vi "Write_ERD_Data_to_File.vi"(0 "refnum in":refnum<file>, 1 "ERD_Always Show":T6, 5 "Redundant Micro":T4, 7 "Version":T5, 9 "ERD Graph  Ind 2":T3, 11 "Error In":errorcluster, 12 "ATC Data":T2, 13 "Algorithm Data":T1) -> (4 "refnum out":refnum<file>, 15 "Error Out":errorcluster)   [LabVIEW 2014]
uses:
  type defs/ERD_Always_Show.ctl
  type defs/Version.ctl
  type defs/Redundant.ctl
  type defs/ATC_Data.ctl
  type defs/Algorithms.ctl
panel:
  # "Wet Load Size"
  # "Dry Load Size"
  # "OOB"
  # "Software Version"
  # "Critical Version"
  # "Non-Critical"
  # "XML Crit Ver"
  # "XML Non-Crit"
  # "Daily Build"
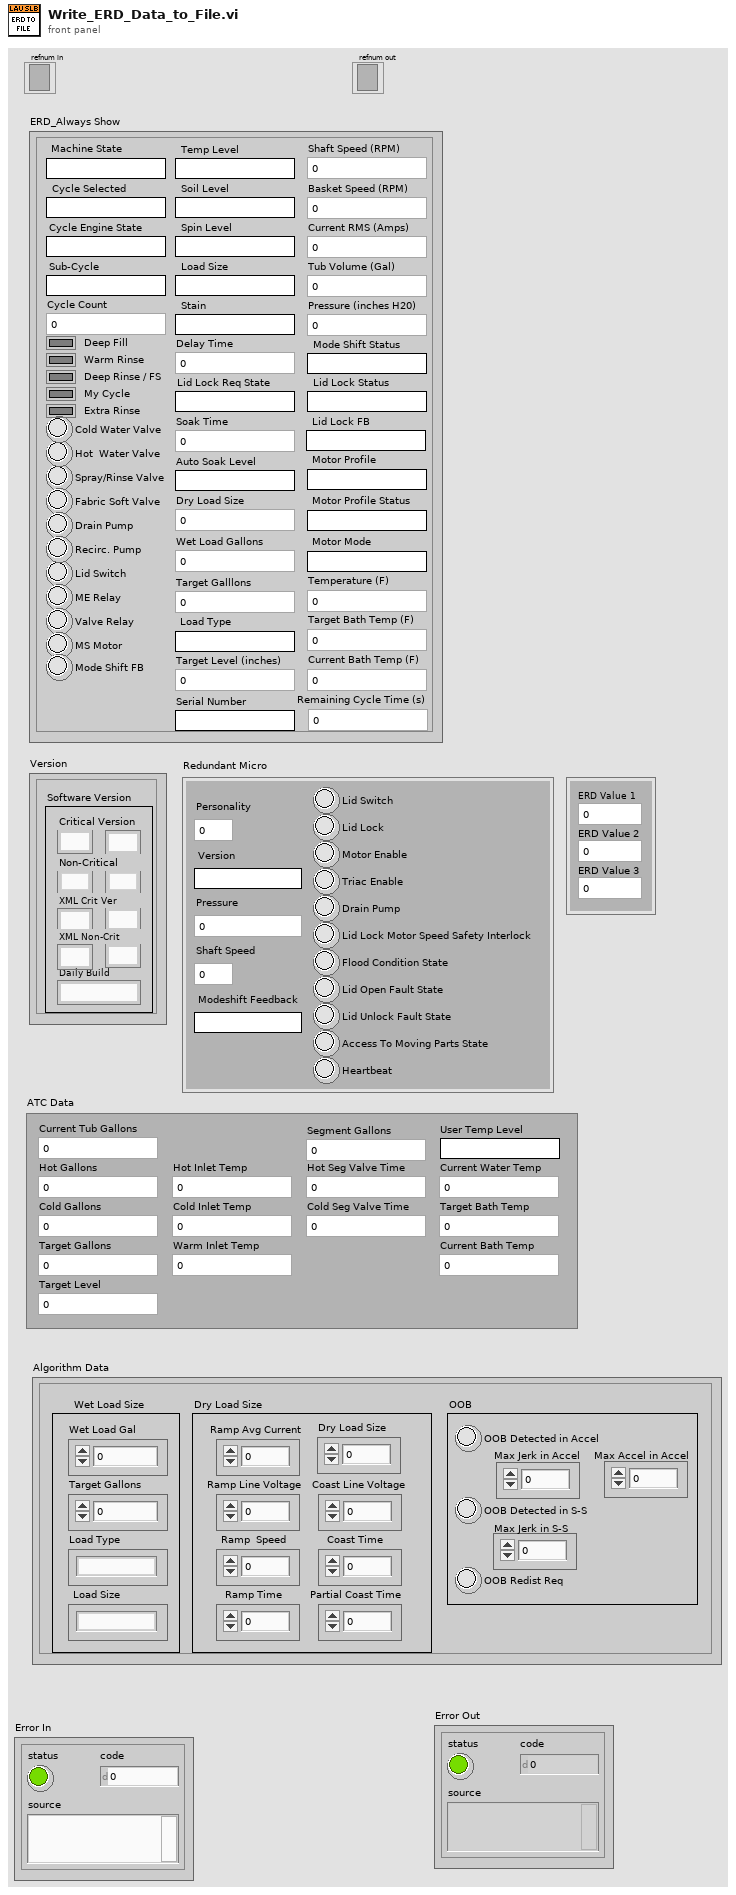
[diagram p1: front panel]
types:
  T1 = typedef "Algorithms.ctl" = cluster{"Wet Load Gal":dbl, "Target Gallons":dbl, "Load Type":string, "Load Size":string, "Coast Time":u16, "Ramp Time":u16, "Ramp  Speed":u16, "Ramp Avg Current":dbl, "OOB Redist Req":bool, "OOB Detected in S-S":bool, "Max Accel in Accel":i32, "Max Jerk in Accel":i32, "Max Jerk in S-S":i32, "OOB Detected in Accel":bool, "Partial Coast Time":u16, "Dry Load Size":dbl, "Ramp Line Voltage ":dbl, "Coast Line Voltage":dbl}
  T2 = typedef "ATC_Data.ctl" = cluster{"Current Tub Gallons":dbl, "Hot Gallons":dbl, "Cold Gallons":dbl, "Target Gallons":dbl, "Current Water Temp":dbl, "Target Level":u32, "Target Bath Temp":dbl, "Current Bath Temp ":dbl, "Cold Inlet Temp":dbl, "Hot Inlet Temp":dbl, "Warm Inlet Temp":dbl, "Hot Seg Valve Time":u16, "Cold Seg Valve Time ":u16, "User Temp Level":string, "Segment Gallons":dbl}
  T3 = cluster{"ERD Value 1":dbl, "ERD Value 2":dbl, "ERD Value 3":dbl}
  T4 = typedef "Redundant.ctl" = cluster{"Version":string, "Personality":u8, "Pressure ":dbl, "Shaft Speed":u16, "Modeshift Feedback":string, "Lid Switch":bool, "Lid Lock":bool, "Triac Enable":bool, "Drain Pump":bool, "Lid Lock Motor Speed Safety Interlock":bool, "Flood Condition State":bool, "Lid Open Fault State":bool, "Access To Moving Parts State":bool, "Heartbeat":bool, "Motor Enable":bool, "Lid Unlock Fault State":bool}
  T5 = typedef "Version.ctl" = cluster{"Critical Major":string, "Critical Minor":string, "Non-Critical Minor":string, "Non-Critical Major":string, "XML Crit Minor":string, "XMLCrit Major":string, "Daily Rev":string, "XML Non-crit Minor":string, "Xml Non-crit Major":string}
  T6 = typedef "ERD_Always_Show.ctl" = cluster{"Basket Speed (RPM)":u16, "Machine State":string, "Tub Volume (Gal)":dbl, "Pressure (inches H20)":dbl, "Lid Switch ":bool, "Current RMS (Amps)":dbl, "Cycle Selected":string, "Lid Lock Status":string, "Mode Shift Status":string, "Spray/Rinse Valve":bool, "Fabric Soft Valve":bool, "Drain Pump":bool, "Recirc. Pump":bool, "Cycle Engine State":string, "Hot  Water Valve":bool, "Cold Water Valve":bool, "Motor Profile":string, "Motor Profile Status":string, "Motor Mode":string, "ME Relay":bool, "Cycle Count":u32, "Deep Rinse / FS":bool, "My Cycle":bool, "Soil Level":string, "Spin Level":string, "Stain":string, "Temp Level":string, "Load Size":string, "Delay Time":u16, "Soak Time":u16, "Deep Fill":bool, "Warm Rinse":bool, "Auto Soak Level":string, "Extra Rinse":bool, "Wet Load Gallons":dbl, "Target Galllons":dbl, "Sub-Cycle":string, "Load Type":string, "Target Level (inches)":u32, "Valve Relay":bool, "Dry Load Size":dbl, "Shaft Speed (RPM) ":u16, "MS Motor":bool, "Mode Shift FB":bool, "Target Bath Temp (F)":dbl, "Temperature (F)":dbl, "Current Bath Temp (F)":dbl, "Lid Lock FB":string, "Lid Lock Req State":string, "Remaining Cycle Time (s)":dbl, "Serial Number":string}
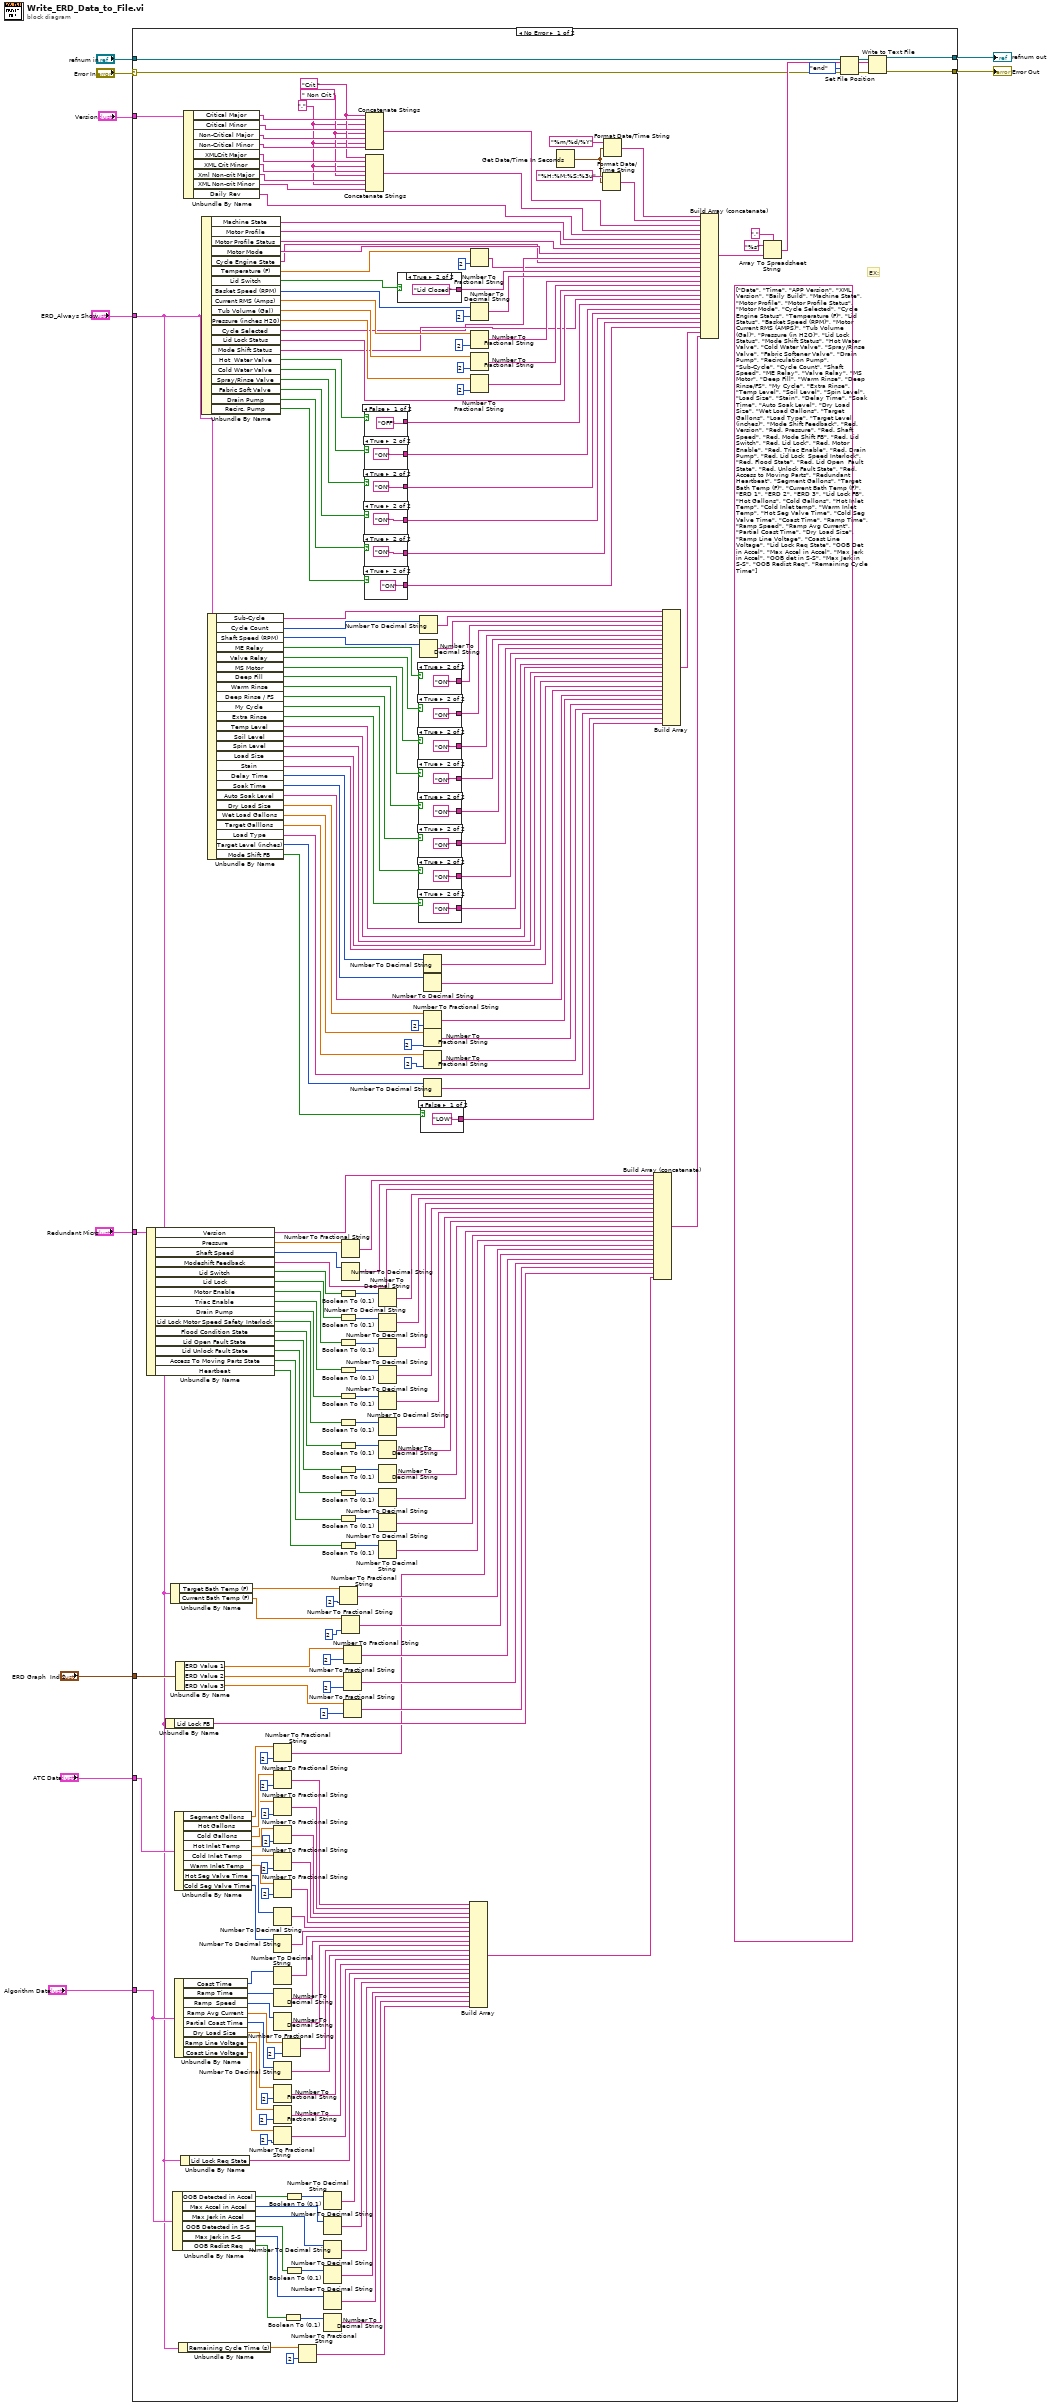
[diagram p0: block diagram]
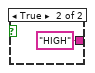
[diagram p2: hidden frame]
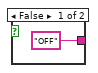
[diagram p3: hidden frame]
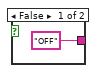
[diagram p4: hidden frame]
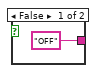
[diagram p5: hidden frame]
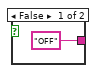
[diagram p6: hidden frame]
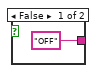
[diagram p7: hidden frame]
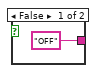
[diagram p8: hidden frame]
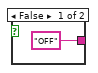
[diagram p9: hidden frame]
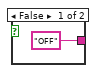
[diagram p10: hidden frame]
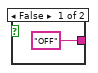
[diagram p11: hidden frame]
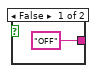
[diagram p12: hidden frame]
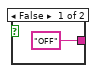
[diagram p13: hidden frame]
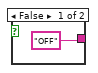
[diagram p14: hidden frame]
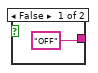
[diagram p15: hidden frame]
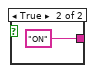
[diagram p16: hidden frame]
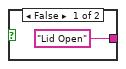
[diagram p17: hidden frame]
diagram:
  n1 = case shown="No Error" "Error In" {
    selector: "Error In" -> [w210 w281]
    tunnel: [w216 w280] -> w8
    tunnel: "ERD_Always Show" -> [w14 _]
    tunnel: "refnum in" -> [w214 w280]
    tunnel: [w211 w281] -> w6
    tunnel: "Version" -> [w152 _]
    tunnel: "Redundant Micro" -> [w135 _]
    tunnel: "ERD Graph  Ind 2" -> [w90 _]
    tunnel: "ATC Data" -> [w82 _]
    tunnel: "Algorithm Data" -> [w49 _]
    frame No Error {
      (unwired) string[] ["Date", "Time", "APP Version", "XML Version", "Baily Build", "Machine State", "Motor Profile", "Motor Profile Status", "Motor Mode", "Cycle Selected", "Cycle Engine Status", "Temperature (F)", "Lid Status", "Basket Speed (RPM)", "Motor Current RMS (AMPS)", "Tub Volume (Gal)", "Pressure (in H2O)", "Lid Lock Status", "Mode Shift Status", "Hot Water Valve", "Cold Water Valve", "Spray/Rinse Valve", "Fabric Softener Valve", "Drain Pump", "Recirculation Pump", "Sub-Cycle", "Cycle Count", "Shaft Speed", "ME Relay", "Valve Relay", "MS Motor", "Deep Fill", "Warm Rinse", "Deep Rinse/FS", "My Cycle", "Extra Rinse", "Temp Level", "Soil Level", "Spin Level", "Load Size", "Stain", "Delay Time", "Soak Time", "Auto Soak Level", "Dry Load Size", "Wet Load Gallons", "Target Gallons", "Load Type", "Target Level (inches)", "Mode Shift Feedback", "Red. Version", "Red. Pressure", "Red. Shaft Speed", "Red. Mode Shift FB", "Red. Lid Switch", "Red. Lid Lock", "Red. Motor Enable", "Red. Triac Enable", "Red. Drain Pump", "Red. Lid Lock  Speed Interlock", "Red. Flood State", "Red. Lid Open  Fault State", "Red. Unlock Fault State", "Red. Access to Moving Parts", "Redundant Heartbeat", "Segment Gallons", "Target Bath Temp (F)", "Current Bath Temp (F)", "ERD 1", "ERD 2", "ERD 3", "Lid Lock FB", "Hot Gallons", "Cold Gallons", "Hot Inlet Temp", "Cold Inlet temp", "Warm Inlet Temp", "Hot Seg Valve Time", "Cold Seg Valve Time", "Coast Time", "Ramp Time", "Ramp Speed", "Ramp Avg Current", "Partial Coast Time", "Dry Load Size", "Ramp Line Voltage", "Coast Line Voltage", "Lid Lock Req State", "OOB Det in Accel", "Max Accel in Accel", "Max Jerk in Accel", "OOB det in S-S", "Max Jerk in S-S", "OOB Redist Req", "Remaining Cycle Time"]
      w144 = " Non Crit " ("element")
      w142 = "." ("element")
      w147 = "Crit " ("element")
      # "EX:"
      n2 = Unbundle By Name(w135) -> ("Version"=w134:string, "Pressure"=w133:dbl, "Shaft Speed"=w131:u16, "Modeshift Feedback"=w129:string, "Lid Switch"=w126:bool, "Lid Lock"=w116:bool, "Motor Enable"=w115:bool, "Triac Enable"=w114:bool, "Drain Pump"=w113:bool, "Lid Lock Motor Speed Safety Interlock"=w112:bool, "Flood Condition State"=w111:bool, "Lid Open Fault State"=w110:bool, "Lid Unlock Fault State"=w108:bool, "Access To Moving Parts State"=w107:bool, "Heartbeat"=w106:bool)
      n3 = Unbundle By Name(w14) -> ("Lid Lock FB"=w83:string)
      n4 = Unbundle By Name(w14) -> ("Target Bath Temp (F)"=w94:dbl, "Current Bath Temp (F)"=w92:dbl)
      n5 = Unbundle By Name(w49) -> ("OOB Detected in Accel"=w47:bool, "Max Accel in Accel"=w45:i32, "Max Jerk in Accel"=w43:i32, "OOB Detected in S-S"=w41:bool, "Max Jerk in S-S"=w40:i32, "OOB Redist Req"=w38:bool)
      n6 = Unbundle By Name(w82) -> ("Segment Gallons"=w16:dbl, "Hot Gallons"=w81:dbl, "Cold Gallons"=w80:dbl, "Hot Inlet Temp"=w79:dbl, "Cold Inlet Temp"=w78:dbl, "Warm Inlet Temp"=w77:dbl, "Hot Seg Valve Time"=w76:u16, "Cold Seg Valve Time"=w75:u16)
      n7 = Unbundle By Name(w49) -> ("Coast Time"=w66:u16, "Ramp Time"=w65:u16, "Ramp  Speed"=w64:u16, "Ramp Avg Current"=w63:dbl, "Partial Coast Time"=w62:u16, "Dry Load Size"=w61:dbl, "Ramp Line Voltage"=w60:dbl, "Coast Line Voltage"=w59:dbl)
      n8 = Unbundle By Name(w90) -> ("ERD Value 1"=w89:dbl, "ERD Value 2"=w88:dbl, "ERD Value 3"=w87:dbl)
      n9 = Unbundle By Name(w14) -> ("Remaining Cycle Time (s)"=w12:dbl)
      n10 = Unbundle By Name(w14) -> ("Lid Lock Req State"=w50:string)
      n11 = Unbundle By Name(w152) -> ("Critical Major"=w151:string, "Critical Minor"=w150:string, "Non-Critical Major"=w149:string, "Non-Critical Minor"=w148:string, "XMLCrit Major"=w146:string, "XML Crit Minor"=w145:string, "Xml Non-crit Major"=w143:string, "XML Non-crit Minor"=w141:string, "Daily Rev"=w136:string)
      n12 = Unbundle By Name(w14) -> ("Machine State"=w246:string, "Motor Profile"=w245:string, "Motor Profile Status"=w204:string, "Motor Mode"=w202:string, "Cycle Engine State"=w198:string, "Temperature (F)"=w203:dbl, "Lid Switch"=w237:bool, "Basket Speed (RPM)"=w238:u16, "Current RMS (Amps)"=w230:dbl, "Tub Volume (Gal)"=w241:dbl, "Pressure (inches H20)"=w240:dbl, "Cycle Selected"=w199:string, "Lid Lock Status"=w229:string, "Mode Shift Status"=w228:string, "Hot  Water Valve"=w227:bool, "Cold Water Valve"=w226:bool, "Spray/Rinse Valve"=w225:bool, "Fabric Soft Valve"=w224:bool, "Drain Pump"=w219:bool, "Recirc. Pump"=w218:bool)
      n13 = Unbundle By Name(w14) -> ("Sub-Cycle"=w196:string, "Cycle Count"=w195:u32, "Shaft Speed (RPM)"=w193:u16, "ME Relay"=w191:bool, "Valve Relay"=w190:bool, "MS Motor"=w189:bool, "Deep Fill"=w188:bool, "Warm Rinse"=w187:bool, "Deep Rinse / FS"=w186:bool, "My Cycle"=w185:bool, "Extra Rinse"=w184:bool, "Temp Level"=w176:string, "Soil Level"=w175:string, "Spin Level"=w174:string, "Load Size"=w173:string, "Stain"=w172:string, "Delay Time"=w171:u16, "Soak Time"=w170:u16, "Auto Soak Level"=w169:string, "Dry Load Size"=w168:dbl, "Wet Load Gallons"=w167:dbl, "Target Galllons"=w166:dbl, "Load Type"=w160:string, "Target Level (inches)"=w158:u32, "Mode Shift FB"=w156:bool)
      n14 = Number To Fractional String(number=w16, precision (6)=i16 2) -> (F-format string=w15:string)  [unwired: 2 in]
      n15 = Number To Fractional String(number=w81, precision (6)=i16 2) -> (F-format string=w74:string)  [unwired: 2 in]
      n16 = Number To Fractional String(number=w80, precision (6)=i16 2) -> (F-format string=w73:string)  [unwired: 2 in]
      n17 = Number To Fractional String(number=w79, precision (6)=i16 2) -> (F-format string=w72:string)  [unwired: 2 in]
      n18 = Number To Fractional String(number=w78, precision (6)=i16 2) -> (F-format string=w71:string)  [unwired: 2 in]
      n19 = Number To Fractional String(number=w77, precision (6)=i16 2) -> (F-format string=w70:string)  [unwired: 2 in]
      n20 = Number To Decimal String(number=w76) -> (decimal integer string=w69:string)  [unwired: 1 in]
      n21 = Number To Decimal String(number=w75) -> (decimal integer string=w68:string)  [unwired: 1 in]
      n22 = Number To Decimal String(number=w66) -> (decimal integer string=w58:string)  [unwired: 1 in]
      n23 = Number To Decimal String(number=w65) -> (decimal integer string=w57:string)  [unwired: 1 in]
      n24 = Number To Decimal String(number=w64) -> (decimal integer string=w56:string)  [unwired: 1 in]
      n25 = Number To Decimal String(number=w62) -> (decimal integer string=w54:string)  [unwired: 1 in]
      n26 = Number To Fractional String(number=w61, precision (6)=i16 2) -> (F-format string=w53:string)  [unwired: 2 in]
      n27 = Number To Fractional String(number=w60, precision (6)=i16 2) -> (F-format string=w52:string)  [unwired: 2 in]
      n28 = Number To Fractional String(number=w59, precision (6)=i16 2) -> (F-format string=w51:string)  [unwired: 2 in]
      n29 = Number To Fractional String(number=w63, precision (6)=i16 2) -> (F-format string=w55:string)  [unwired: 2 in]
      n30 = Boolean To (0,1)(Boolean=w38) -> (0, 1=w39:i16)
      n31 = Boolean To (0,1)(Boolean=w47) -> (0, 1=w48:i16)
      n32 = Boolean To (0,1)(Boolean=w41) -> (0, 1=w42:i16)
      n33 = Number To Fractional String(number=w12, precision (6)=i16 2) -> (F-format string=w11:string)  [unwired: 2 in]
      n34 = Number To Decimal String(number=w48) -> (decimal integer string=w46:string)  [unwired: 1 in]
      n35 = Number To Decimal String(number=w45) -> (decimal integer string=w44:string)  [unwired: 1 in]
      n36 = Number To Decimal String(number=w43) -> (decimal integer string=w37:string)  [unwired: 1 in]
      n37 = Number To Decimal String(number=w42) -> (decimal integer string=w36:string)  [unwired: 1 in]
      n38 = Number To Decimal String(number=w40) -> (decimal integer string=w35:string)  [unwired: 1 in]
      n39 = Number To Decimal String(number=w39) -> (decimal integer string=w34:string)  [unwired: 1 in]
      n40 = Boolean To (0,1)(Boolean=w126) -> (0, 1=w128:i16)
      n41 = Boolean To (0,1)(Boolean=w116) -> (0, 1=w125:i16)
      n42 = Boolean To (0,1)(Boolean=w115) -> (0, 1=w124:i16)
      n43 = Boolean To (0,1)(Boolean=w114) -> (0, 1=w123:i16)
      n44 = Boolean To (0,1)(Boolean=w113) -> (0, 1=w122:i16)
      n45 = Boolean To (0,1)(Boolean=w112) -> (0, 1=w121:i16)
      n46 = Boolean To (0,1)(Boolean=w111) -> (0, 1=w120:i16)
      n47 = Boolean To (0,1)(Boolean=w110) -> (0, 1=w119:i16)
      n48 = Boolean To (0,1)(Boolean=w108) -> (0, 1=w118:i16)
      n49 = Boolean To (0,1)(Boolean=w107) -> (0, 1=w117:i16)
      n50 = Boolean To (0,1)(Boolean=w106) -> (0, 1=w109:i16)
      n51 = Number To Fractional String(number=w94, precision (6)=i16 2) -> (F-format string=w93:string)  [unwired: 2 in]
      n52 = Number To Fractional String(number=w92, precision (6)=i16 2) -> (F-format string=w91:string)  [unwired: 2 in]
      n53 = Number To Fractional String(number=w133) -> (F-format string=w132:string)  [unwired: 3 in]
      n54 = Number To Decimal String(number=w131) -> (decimal integer string=w130:string)  [unwired: 1 in]
      n55 = Number To Fractional String(number=w89, precision (6)=i16 2) -> (F-format string=w86:string)  [unwired: 2 in]
      n56 = Number To Fractional String(number=w88, precision (6)=i16 2) -> (F-format string=w85:string)  [unwired: 2 in]
      n57 = Number To Fractional String(number=w87, precision (6)=i16 2) -> (F-format string=w84:string)  [unwired: 2 in]
      n58 = case shown="False" w227 {
        tunnel: ["OFF" "ON"] -> w223
        frame False {
        }
        frame True {
        }
      }
      n59 = case shown="True" w226 {
        tunnel: ["OFF" "ON"] -> w200
        frame False {
        }
        frame True {
        }
      }
      n60 = case shown="True" w225 {
        tunnel: ["OFF" "ON"] -> w222
        frame False {
        }
        frame True {
        }
      }
      n61 = case shown="True" w224 {
        tunnel: ["OFF" "ON"] -> w221
        frame False {
        }
        frame True {
        }
      }
      n62 = case shown="True" w219 {
        tunnel: ["OFF" "ON"] -> w220
        frame False {
        }
        frame True {
        }
      }
      n63 = case shown="True" w218 {
        tunnel: ["OFF" "ON"] -> w201
        frame False {
        }
        frame True {
        }
      }
      n64 = Concatenate Strings(w147, w151, w142, w150, w144, w149, w142, w148) -> (w138:string)
      n65 = Concatenate Strings(w147, w146, w142, w145, w144, w143, w142, w141) -> (w137:string)
      n66 = Number To Decimal String(number=w128) -> (decimal integer string=w127:string)  [unwired: 1 in]
      n67 = Number To Decimal String(number=w125) -> (decimal integer string=w105:string)  [unwired: 1 in]
      n68 = Number To Decimal String(number=w124) -> (decimal integer string=w104:string)  [unwired: 1 in]
      n69 = Number To Decimal String(number=w123) -> (decimal integer string=w103:string)  [unwired: 1 in]
      n70 = Number To Decimal String(number=w122) -> (decimal integer string=w102:string)  [unwired: 1 in]
      n71 = Number To Decimal String(number=w121) -> (decimal integer string=w101:string)  [unwired: 1 in]
      n72 = Number To Decimal String(number=w120) -> (decimal integer string=w100:string)  [unwired: 1 in]
      n73 = Number To Decimal String(number=w119) -> (decimal integer string=w99:string)  [unwired: 1 in]
      n74 = Number To Decimal String(number=w118) -> (decimal integer string=w98:string)  [unwired: 1 in]
      n75 = Number To Decimal String(number=w117) -> (decimal integer string=w97:string)  [unwired: 1 in]
      n76 = Number To Decimal String(number=w109) -> (decimal integer string=w96:string)  [unwired: 1 in]
      n77 = case shown="True" w237 {
        tunnel: ["Lid Open" "Lid Closed"] -> w236
        frame False {
        }
        frame True {
        }
      }
      n78 = case shown="True" w191 {
        tunnel: ["OFF" "ON"] -> w183
        frame False {
        }
        frame True {
        }
      }
      n79 = case shown="True" w190 {
        tunnel: ["OFF" "ON"] -> w182
        frame False {
        }
        frame True {
        }
      }
      n80 = case shown="True" w189 {
        tunnel: ["OFF" "ON"] -> w181
        frame False {
        }
        frame True {
        }
      }
      n81 = case shown="True" w188 {
        tunnel: ["OFF" "ON"] -> w180
        frame False {
        }
        frame True {
        }
      }
      n82 = case shown="True" w187 {
        tunnel: ["OFF" "ON"] -> w179
        frame False {
        }
        frame True {
        }
      }
      n83 = case shown="True" w186 {
        tunnel: ["OFF" "ON"] -> w178
        frame False {
        }
        frame True {
        }
      }
      n84 = case shown="True" w185 {
        tunnel: ["OFF" "ON"] -> w177
        frame False {
        }
        frame True {
        }
      }
      n85 = case shown="True" w184 {
        tunnel: ["OFF" "ON"] -> w154
        frame False {
        }
        frame True {
        }
      }
      n86 = Number To Decimal String(number=w195) -> (decimal integer string=w194:string)  [unwired: 1 in]
      n87 = Number To Decimal String(number=w193) -> (decimal integer string=w192:string)  [unwired: 1 in]
      n88 = case shown="False" w156 {
        tunnel: ["LOW" "HIGH"] -> w155
        frame False {
        }
        frame True {
        }
      }
      n89 = Number To Decimal String(number=w171) -> (decimal integer string=w165:string)  [unwired: 1 in]
      n90 = Number To Decimal String(number=w170) -> (decimal integer string=w164:string)  [unwired: 1 in]
      n91 = Number To Fractional String(number=w168, precision (6)=i16 2) -> (F-format string=w163:string)  [unwired: 2 in]
      n92 = Number To Fractional String(number=w167, precision (6)=i16 2) -> (F-format string=w162:string)  [unwired: 2 in]
      n93 = Number To Fractional String(number=w166, precision (6)=i16 2) -> (F-format string=w161:string)  [unwired: 2 in]
      n94 = Number To Decimal String(number=w158) -> (decimal integer string=w159:string)  [unwired: 1 in]
      n95 = Build Array(w74, w73, w72, w71, w70, w69, w68, w58, w57, w56, w55, w54, w53, w52, w51, w50, w46, w44, w37, w36, w35, w34, w11) -> (w67:string[])
      n96 = Number To Fractional String(number=w203, precision (6)=i16 2) -> (F-format string=w197:string)  [unwired: 2 in]
      n97 = Number To Decimal String(number=w238, width (-)=i16 2 ("precision (6)")) -> (decimal integer string=w235:string)
      n98 = Number To Fractional String(number=w230, precision (6)=i16 2) -> (F-format string=w234:string)  [unwired: 2 in]
      n99 = Number To Fractional String(number=w241, precision (6)=i16 2) -> (F-format string=w233:string)  [unwired: 2 in]
      n100 = Number To Fractional String(number=w240, precision (6)=i16 2) -> (F-format string=w232:string)  [unwired: 2 in]
      n101 = Get Date/Time In Seconds() -> (seconds since 1Jan1904=w206:timestamp)
      n102 = Format Date/Time String(time format string (%c)="%H:%M:%S:%3u", seconds (now)=w206) -> (date/time string=w139:string)  [unwired: 1 in]
      n103 = Format Date/Time String(time format string (%c)="%m/%d/%Y", seconds (now)=w206) -> (date/time string=w140:string)  [unwired: 1 in]
      n104 = Build Array (concatenate)(w134, w132, w130, w129, w127, w105, w104, w103, w102, w101, w100, w99, w98, w97, w96, w15, w93, w91, w86, w85, w84, w83, w67) -> (w95:string[])
      n105 = Build Array(w196, w194, w192, w183, w182, w181, w180, w179, w178, w177, w154, w176, w175, w174, w173, w172, w165, w164, w169, w163, w162, w161, w160, w159, w155) -> (w157:string[])
      n106 = Build Array (concatenate)(w140, w139, w138, w137, w136, w246, w245, w204, w202, w199, w198, w197, w236, w235, w234, w233, w232, w229, w228, w223, w200, w222, w221, w220, w201, w157, w95) -> (w205:string[])
      n107 = Array To Spreadsheet String(delimiter (Tab)=",", array=w205, 3:"%s" ("format string")) -> (spreadsheet string=w217:string)
      n108 = Set File Position(refnum=w214, from (0:start)=enum16{"start", "end", "current"}."end", error in=w210) -> (refnum out=w213:refnum<file>, error out=w212:errorcluster)  [unwired: 1 in]
      n109 = Write to Text File(file (use dialog)=w213, text=w217, error in=w212) -> (refnum out=w216:refnum<file>, error out=w211:errorcluster)  [unwired: 1 in, 1 out]
    }
    frame Error {
    }
  }
  "Error Out" <- w6
  "refnum out" <- w8
